vi "findPath.vi"(8 "error in (no error)":errorcluster, 9 "Path":path, 11 "ExperimentRunner in":refnum<class "ExperimentRunner.lvclass">) -> (0 "error out":errorcluster, 1 "index of element":i32, 3 "ExperimentRunner out":refnum<class "ExperimentRunner.lvclass">)   [LabVIEW 2009, in "Views.lvlib" / "ExperimentControl.lvlib" / "ExperimentRunner.lvclass"]
uses:
  ExperimentRunner.lvclass
  ExperimentRunner.lvclass/ExperimentRunner.ctl
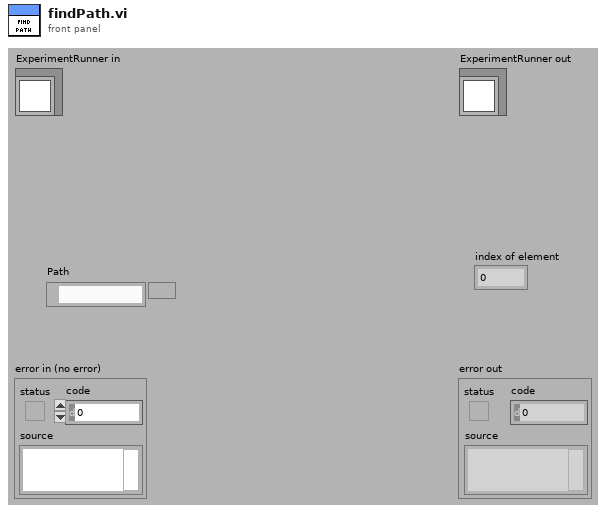
[diagram p1: front panel]
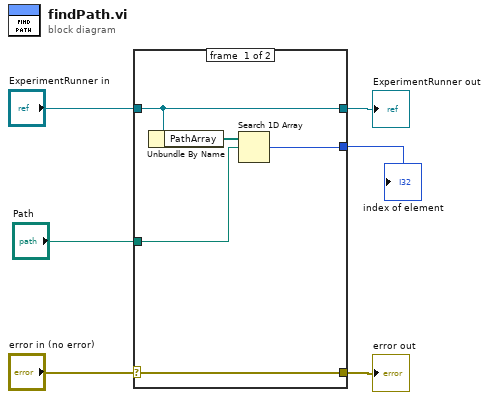
[diagram p0: block diagram]
diagram:
  n1 = case shown="No Error" "error in (no error)" {
    selector: "error in (no error)" -> [w11 w13]
    tunnel: [w11 w13] -> w5
    tunnel: [w10 w12] -> w3
    tunnel: "ExperimentRunner in" -> [w10 w12]
    tunnel: "Path" -> [w8 _]
    tunnel: [w7 _] -> w1
    frame #0 {
      n2 = Unbundle By Name(w10) -> ("PathArray"=w9:path[])
      n3 = Search 1D Array(1D array=w9, element=w8) -> (index of element=w7:i32)  [unwired: 1 in]
    }
    frame #1 {
    }
  }
  "error out" <- w5
  "ExperimentRunner out" <- w3
  "index of element" <- w1
